vi "niRFUtil MT UTIL Integer Rate Interpolation (Complex SGL).vi"(4 "flush buffers? (F)":bool, 6 "reset? (T)":bool=TRUE, 9 "interpolation factor":i32=10, 11 "input[]":csg[](array[numeric])) -> (3 "output[]":csg[](array[numeric]), 5 "filter coefficients out[]":sgl[](array[numeric]))   [LabVIEW 2015, in "niRFUtil.lvlib"]
uses:
  niRFUtil.lvlib
  Includes/niRFUtil MT INC Integer Interpolator State (Complex SGL).ctl
  niRFAMT.dll
panel:
  in  "default state":T1
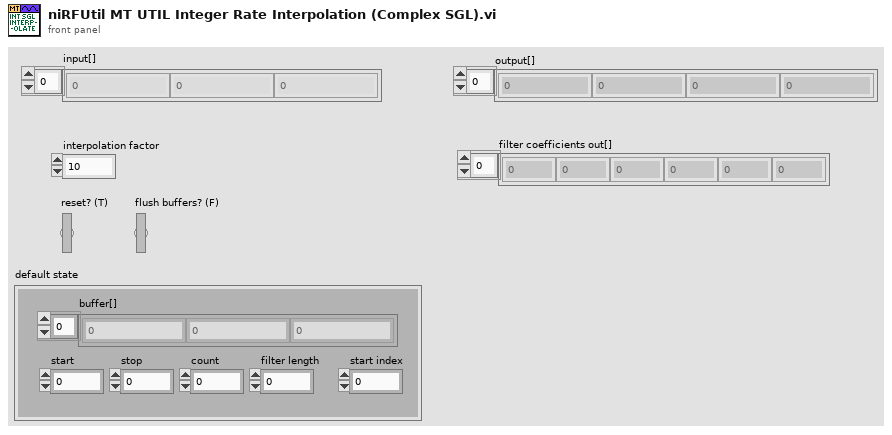
[diagram p1: front panel]
types:
  T1 = typedef "niRFUtil.lvlib/niRFUtil MT INC Integer Interpolator State (Complex SGL).ctl" = cluster{"buffer[]":csg[], "start":i32, "stop":i32, "count":i32, "filter length":i32, "start index":i32}
  T2 = typedef "niRFUtil.lvlib/niRFUtil INC Real Array.ctl" = sgl[]
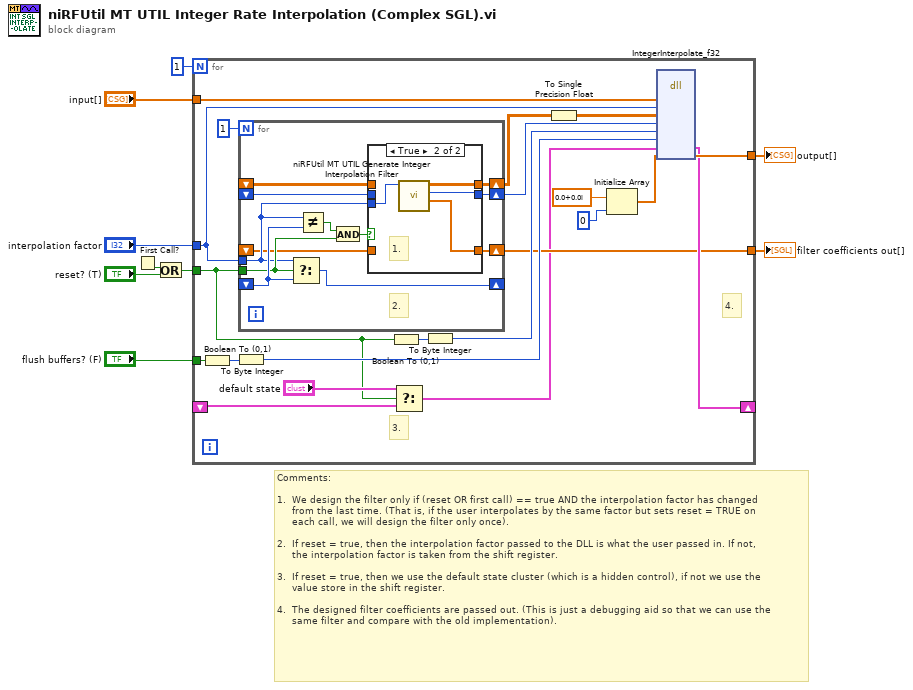
[diagram p0: block diagram]
diagram:
  # "Comments:\n\n1.  We design the filter only if (reset OR first call) == true AND the interpolation factor has changed\n     from the last time. (That is, if the user interpolates by the same factor but sets reset = TRUE on\n     each call, we will design the filter only once).\n\n2.  If reset = true, then the interpolation factor passed to the DLL is what the user passed in. If not,\n     the interpolation factor is taken from the shift register.\n\n3.  If reset = true, then we use the default state cluster (which is a hidden control), if not we use the\n     value store in the shift register.\n\n4.  The designed filter coefficients are passed out. (This is just a debugging aid so that we can use the\n     same filter and compare with the old implementation)."
  n1 = First Call?() -> (First Call?: T/F=w7:bool)
  n2 = Or(x=w7, y="reset? (T)") -> (x .or. y?=w6:bool)
  n3 = for {
    N: 1 -> [_]
    tunnel: "interpolation factor" -> [w28]
    tunnel: w6 -> [w12]
    shift-right: [w17] -> _
    shift-left: _ -> [w13]
    tunnel: "input[]" -> [w29]
    tunnel: "flush buffers? (F)" -> [w23]
    tunnel: [w18] -> w2
    tunnel: [w16] -> w1
    # "4."
    # "3."
    n4 = Boolean To (0,1)(Boolean=w23) -> (0, 1=w24:i16)
    n5 = To Byte Integer(number=w24) -> (8bit integer=w22:i8)
    n6 = for {
      N: 1 -> [_]
      shift-right: [w42] -> _
      shift-left: _ -> [w40]
      tunnel: w12 -> [w38]
      tunnel: w28 -> [w34]
      shift-right: [w41] -> w10
      shift-left: _ -> [w37]
      shift-right: [w36] -> w27
      shift-left: _ -> [w35]
      shift-right: [w33] -> w16
      shift-left: _ -> [w32]
      # "2."
      n7 = Select(t=w34, s=w38, f=w40) -> (s? t:f=w42:i32)
      n8 = Not Equal?(x=w34, y=w40) -> (x != y?=w39:bool)
      n9 = And(x=w39, y=w38) -> (x .and. y?=w31:bool)
      n10 = case shown="True" w31 {
        tunnel: [w45 w49] -> w41
        tunnel: w37 -> [w45 _]
        tunnel: [w44 w48] -> w36
        tunnel: w35 -> [w44 _]
        tunnel: w34 -> [_ w47]
        tunnel: [w43 w46] -> w33
        tunnel: w32 -> [w43 _]
        frame False {
        }
        frame True {
          # "1."
          n11 = call "niRFUtil MT UTIL Generate Integer Interpolation Filter.vi"("interpolation factor"=w47) -> ("filter coefficients out"=w46:T2, "total length"=w48:i32, "polyphase filter out (2D)"=w49:sgl[][])  [unwired: 7 in, 1 out]
        }
      }
    }
    n12 = Boolean To (0,1)(Boolean=w12) -> (0, 1=w26:i16)
    n13 = Select(t="default state", s=w12, f=w13) -> (s? t:f=w15:T1)
    n14 = To Byte Integer(number=w26) -> (8bit integer=w25:i8)
    n15 = To Single Precision Float(number=w10) -> (single precision float=w11:sgl[][])
    n16 = Initialize Array(csg 0.0+0.0i ("element"), 0 ("dimension size")) -> (w19:csg[])
    n17 = dll-call lib="C:/Perforce/semoore-sales/Customers/NATI-3813/Noise Floor/LV Filters/ParallelComplexFilterRFUtil/niRFUtil/MT/Utilities/niRFAMT.*" fn="IntegerInterpolate_f32"("input"=w29, "interpolationFactor"=w28, "filter"=w11, "filterLength"=w27, "reset"=w25, "flush"=w22, "state"=w15, "output"=w19) -> ("state"=w17:T1, "output"=w18:csg[])  [unwired: 9 in, 3 out]
  }
  "output[]" <- w2
  "filter coefficients out[]" <- w1
